vi "Button Definition JSON File Read Error.vi"(10 "error code":i32, 11 "Button Def JSON":path) -> (0 "error out":errorcluster)   [LabVIEW 2020, in "Navigation.lvlib" / "Button Manager.lvclass"]
doc: "____\nHAMPEL SOFTWARE ENGINEERING v2.6.0 (2023-12-19 10:54)"
uses:
  Button Manager.lvclass
  Button Manager.lvclass/Button Manager.ctl
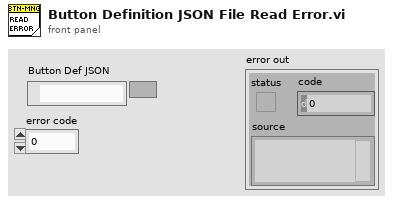
[diagram p1: front panel]
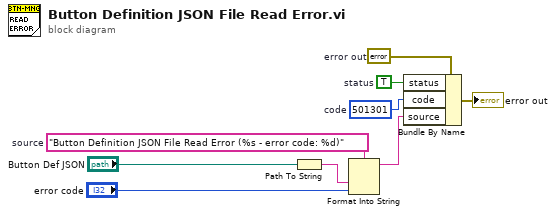
[diagram p0: block diagram]
diagram:
  w5 = "Button Definition JSON File Read Error (%s - error code: %d)"  # source
  w6 = 501301  # code
  w7 = TRUE  # status
  w9 = errorcluster {"status"=FALSE, "code"=0, "source"=""}  # error out
  n1 = Path To String(path="Button Def JSON") -> (string=w2:string)
  n2 = Format Into String(format string=w5, w2, "error code") -> (resulting string=w1:string)  [unwired: 2 in, 1 out]
  n3 = Bundle By Name(cluster=w9, "status"=w7, "code"=w6, "source"=w1) -> (→"error out":errorcluster)
